vi "Service Stop Handler.vi"(8 "error in (no error)":errorcluster, 10 "Stop Button [ref]":refnum<vi>, 11 "MeasurementServiceV1 in":refnum<class "MeasurementServiceV1.lvclass">) -> (0 "error out":errorcluster, 3 "MeasurementServiceV1 out":refnum<class "MeasurementServiceV1.lvclass">)   [LabVIEW 2020, in "MeasurementLink Measurement Server.lvlib" / "MeasurementServiceV1.lvclass"]
uses:
  MeasurementServiceV1.lvclass
  MeasurementServiceV1.lvclass/MeasurementServiceV1.ctl
  MeasurementLink Measurement Server Internal/RPC Service/MeasurementService/MeasurementService.lvclass
  C:/Program Files/National Instruments/LabVIEW 2020/vi.lib/gRPC/LabVIEW gRPC Servicer/ServiceBase/ServiceBase.lvclass
  IMeasurementService/IMeasurementService.lvclass
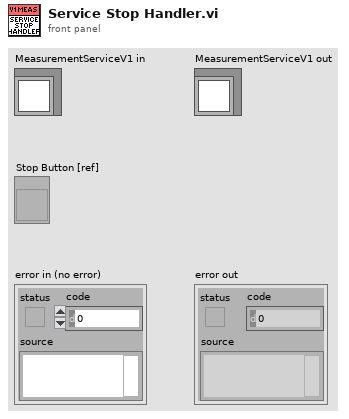
[diagram p1: front panel]
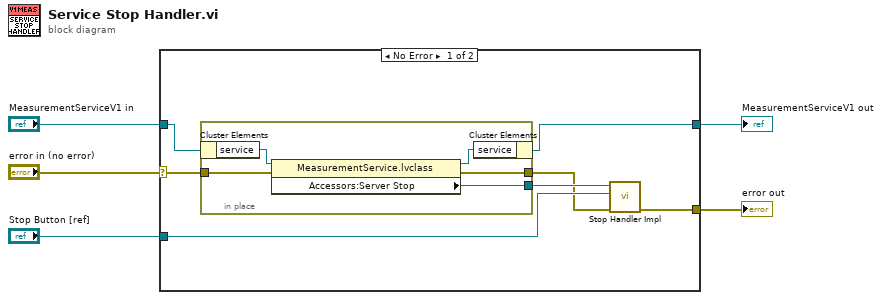
[diagram p0: block diagram]
diagram:
  n1 = case shown="No Error" "error in (no error)" {
    selector: "error in (no error)" -> [w11 w19]
    tunnel: [w10 w19] -> w4
    tunnel: [w9 w18] -> w2
    tunnel: "MeasurementServiceV1 in" -> [w12 w18]
    tunnel: "Stop Button [ref]" -> [w8 _]
    frame No Error {
      n2 = in-place {
        in-place-border: [w15] -> w7
        in-place-border: w11 -> [w14]
        in-place-border: [w13] -> w6
        n3 = in-place-cluster #1(w12) -> ("service"=w17:refnum<class "MeasurementService.lvclass">)
        n4 = property class="MeasurementService.lvclass"(reference=w17, error in=w14) -> (reference out=w16:refnum<class "MeasurementService.lvclass">, error out=w13:errorcluster, "Accessors:Server Stop"=w15:refnum<user-event>)
        n5 = in-place-cluster #1("service"=w16) -> (w9:refnum<class "MeasurementServiceV1.lvclass">)
      }
      n6 = call "Stop Handler Impl.vi"("error in (no error)"=w6, "Stop Button [ref]"=w8, "User Event in"=w7) -> ("error out"=w10:errorcluster)  [unwired: 8 in]
    }
    frame Error {
    }
  }
  "error out" <- w4
  "MeasurementServiceV1 out" <- w2
